vi "Set Metadata.vi"(8 "error in (no error)":errorcluster, 9 "Sphere Indicator":T5=enum."Insulated Sphere", 10 "Analyzer Choice":T3, 11 "Instrument Control \nSwitches":T4) -> (0 "error out":errorcluster, 2 "Metadata Cluster Out":T2)   [LabVIEW 2014, in "Metadata.lvlib"]
uses:
  Metadata.lvlib
  avantesSpectrometer/Acquisition/Sphere Indicator.ctl
  controls/Instrument Control Switches.ctl
  controls/Analyzer Choice.ctl
  Metadata Control.ctl
  Metadata Cluster.ctl
  avantesSpectrometer/AvaSpec.lvlib
panel:
  in  "Tab Control":enum32{"Naked Sphere", "Insulated Sphere"}(tab)
  in  "Metadata Fields Naked Sphere":T1
  in  "Metadata Fields Insualted Sphere":T1
  in  "Output Path":path
  in  "Cancel":bool
  in  "Ready?":bool
  # "Fill out the follow data fields for each test. An error will be thrown if any data fields are missing.\nNew parameters for data fields can be added by right clicking, hitting \"properties\", then \"edit items\""
  # "Off screen"
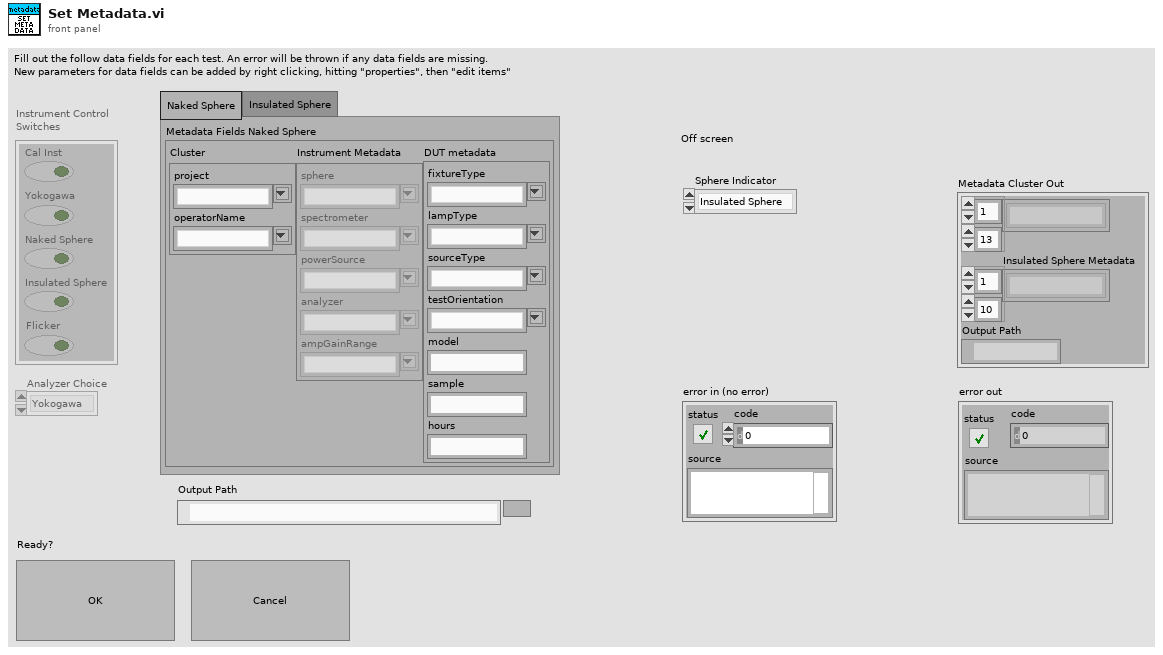
[diagram p1: front panel]
types:
  T1 = typedef "Metadata Control.ctl" = cluster{"Cluster":cluster{"project":string, "operatorName":string}, "Instrument Metadata":cluster{"sphere":string, "spectrometer":string, "powerSource":string, "analyzer":string, "ampGainRange":string}, "DUT metadata":cluster{"fixtureType":string, "lampType":string, "sourceType":string, "testOrientation":string, "model":string, "sample":string, "hours":string}}
  T2 = typedef "Metadata Cluster.ctl" = cluster{"Naked Sphere Metadata":string[][], "Insulated Sphere Metadata":string[][], "Output Path":path}
  T3 = typedef "Analyzer Choice.ctl" = enum16{"Yokogawa", "Cal Inst"}
  T4 = typedef "Instrument Control Switches.ctl" = cluster{"Cal Inst":bool, "Yokogawa":bool, "Naked Sphere":bool, "Insulated Sphere":bool, "Flicker":bool}
  T5 = typedef "AvaSpec.lvlib/Sphere Indicator.ctl" = enum16{"Naked Sphere", "Insulated Sphere"}
  T6 = enum8{"Enabled", "Disabled", "Disabled and Grayed Out"}
  T7 = cluster{"sphere":string, "spectrometer":string, "powerSource":string, "analyzer":string, "ampGainRange":string}
  T8 = cluster{"fixtureType":string, "lampType":string, "sourceType":string, "testOrientation":string, "model":string, "sample":string, "hours":string}
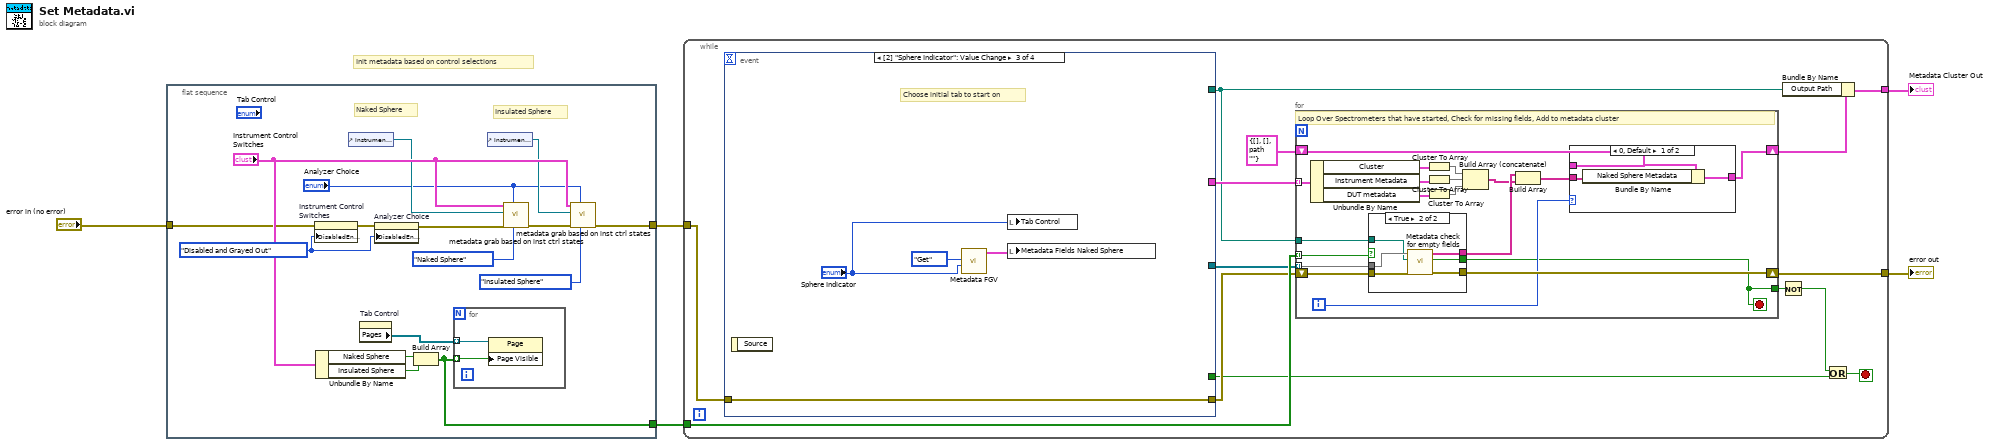
[diagram p0: block diagram]
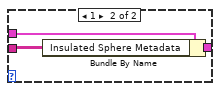
[diagram p2: hidden frame]
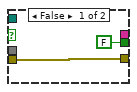
[diagram p3: hidden frame]
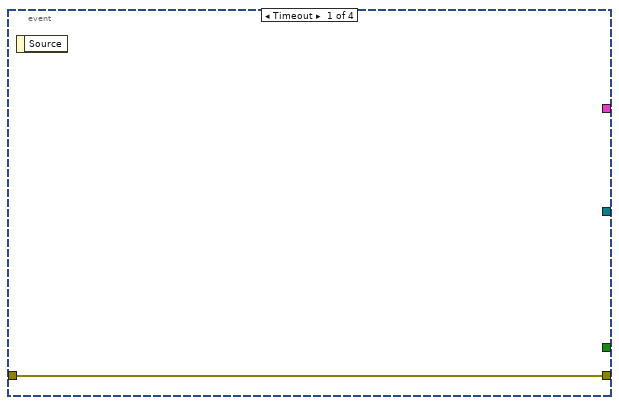
[diagram p4: hidden frame]
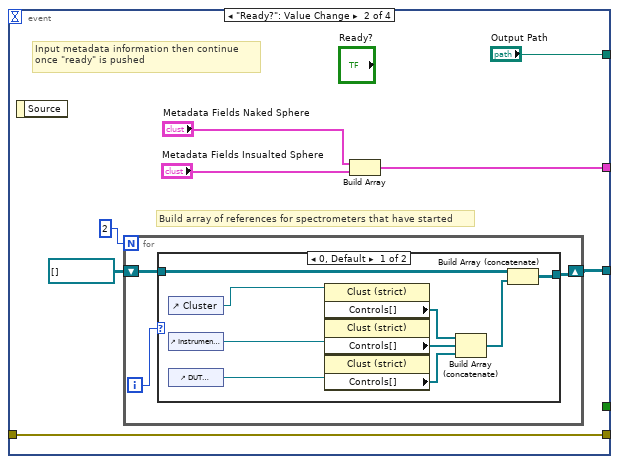
[diagram p5: hidden frame]
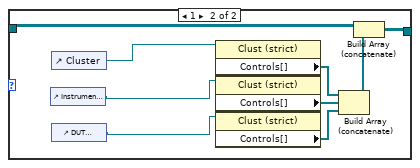
[diagram p6: hidden frame]
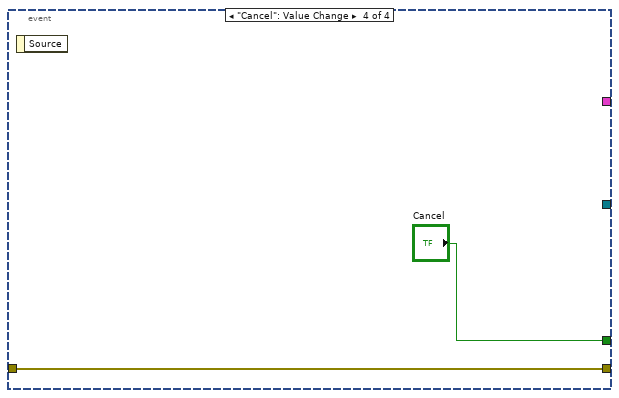
[diagram p7: hidden frame]
diagram:
  # "Init metadata based on control selections"
  n1 = flat-sequence {
    tunnel: [w20] -> w4
    tunnel: [w13] -> w3
    tunnel: "error in (no error)" -> [w9]
    frame #0 {
      w6 = T6."Disabled and Grayed Out" ("Disabled")
      # "Insulated Sphere"
      # "Naked Sphere"
      n2 = property on="Instrument Control \nSwitches" class="Clust (strict)"(error in=w9, "DisabledEnum"=w6) -> (error out=w8:errorcluster)  [unwired: 1 in, 1 out]
      n3 = Unbundle By Name("Instrument Control \nSwitches") -> ("Naked Sphere"=w16:bool, "Insulated Sphere"=w15:bool)
      n4 = control-ref of="Instrument Metadata"() -> (w12:refnum<vi>)
      n5 = property on="Tab Control" class="TabCtl (strict)"() -> ("Pages"=w14:refnum<vi>[])  [unwired: 2 in, 2 out]
      n6 = property on="Analyzer Choice" class="Enum (strict)"(error in=w8, "DisabledEnum"=w6) -> (error out=w7:errorcluster)  [unwired: 1 in, 1 out]
      n7 = Build Array(w16, w15) -> (w13:bool[])
      n8 = for {
        tunnel: w13 -> [w22] mode=indexing
        tunnel: w14 -> [w23] mode=indexing
        n9 = property class="Page"(reference=w23, "Page Visible"=w22) -> ()  [unwired: 1 in, 2 out]
      }
      n10 = control-ref of="Instrument Metadata"() -> (w11:refnum<vi>)
      n11 = call "metadata grab based on inst ctrl states.vi"("Sphere Indicator"=Sphere_Indicator."Naked Sphere" ("Sphere Indicator 2"), "Analyzer Choice"="Analyzer Choice", "error in (no error)"=w7, "Instrument Metadata"=w12, "Instrument Control \nSwitches"="Instrument Control \nSwitches") -> ("error out"=w21:errorcluster)  [unwired: 6 in]
      n12 = call "metadata grab based on inst ctrl states.vi"("Sphere Indicator"=Sphere_Indicator."Insulated Sphere" ("Sphere Indicator 2"), "Analyzer Choice"="Analyzer Choice", "error in (no error)"=w21, "Instrument Metadata"=w11, "Instrument Control \nSwitches"="Instrument Control \nSwitches") -> ("error out"=w20:errorcluster)  [unwired: 6 in]
    }
  }
  n13 = while {
    tunnel: w4 -> [w37]
    tunnel: [w36] -> w1
    tunnel: w3 -> [w34]
    tunnel: [w29] -> w2
    stop <- w35 stop-if-true
    n14 = event shown="[2] \"Sphere Indicator\": Value Change" {
      selector: _ -> [_ _ _ _]
      dyn-events: _ -> [_ _ _ _]
      timeout: _ -> [_ _ _ _]
      tunnel: w37 -> [w71 w72 w102 w106]
      tunnel: [w71 w72 w102 w106] -> w31
      tunnel: [_ _ _ "Cancel"] -> w28
      tunnel: [_ "Output Path" _ _] -> w25
      tunnel: [_ w78 _ _] -> w32
      tunnel: [_ w74 _ _] -> w33
      event Timeout {
        n15 = event-data() -> ()  [unwired: 1 in, 1 out]
      }
      event "Ready?": Value Change {
        # "Build array of references for spectrometers that have started"
        # "Input metadata information then continue\nonce \"ready\" is pushed"
        n16 = event-data() -> ()  [unwired: 1 in, 1 out]
        n17 = for {
          N: 2 -> [_]
          shift-right: [w80] -> w78
          shift-left: refnum<vi>[][] [] -> [w81]
          i -> [w82]
          n18 = case shown="0, Default" w82 {
            tunnel: [w84 w93] -> w80
            tunnel: w81 -> [w83 w92]
            frame 0, Default {
              n19 = control-ref of="Cluster"() -> (w88:refnum<vi>)
              n20 = control-ref of="Instrument Metadata"() -> (w87:refnum<vi>)
              n21 = control-ref of="DUT metadata"() -> (w86:refnum<vi>)
              n22 = property class="Clust (strict)"(reference=w88) -> ("Controls[]"=w91:refnum<vi>[])  [unwired: 1 in, 2 out]
              n23 = property class="Clust (strict)"(reference=w87) -> ("Controls[]"=w90:refnum<vi>[])  [unwired: 1 in, 2 out]
              n24 = property class="Clust (strict)"(reference=w86) -> ("Controls[]"=w89:refnum<vi>[])  [unwired: 1 in, 2 out]
              n25 = Build Array (concatenate)(w91, w90, w89) -> (w85:refnum<vi>[])
              n26 = Build Array (concatenate)(w83, w85) -> (w84:refnum<vi>[][])
            }
            frame 1 {
              n27 = control-ref of="Instrument Metadata"() -> (w95:refnum<vi>)
              n28 = control-ref of="Cluster"() -> (w96:refnum<vi>)
              n29 = control-ref of="DUT metadata"() -> (w94:refnum<vi>)
              n30 = property class="Clust (strict)"(reference=w96) -> ("Controls[]"=w100:refnum<vi>[])  [unwired: 1 in, 2 out]
              n31 = property class="Clust (strict)"(reference=w95) -> ("Controls[]"=w99:refnum<vi>[])  [unwired: 1 in, 2 out]
              n32 = property class="Clust (strict)"(reference=w94) -> ("Controls[]"=w98:refnum<vi>[])  [unwired: 1 in, 2 out]
              n33 = Build Array (concatenate)(w100, w99, w98) -> (w97:refnum<vi>[])
              n34 = Build Array (concatenate)(w92, w97) -> (w93:refnum<vi>[][])
            }
          }
        }
        n35 = Build Array("Metadata Fields Naked Sphere", "Metadata Fields Insualted Sphere") -> (w74:T1[])
      }
      event Value Change {
        # "Choose initial tab to start on"
        n36 = event-data() -> ()  [unwired: 1 in, 1 out]
        n37 = call "Metadata FGV.vi"("Sphere Indicator"="Sphere Indicator", "Control"=enum16{"Get", "Set"}."Get") -> ("Metadata Fields Out"=w103:T1)  [unwired: 9 in]
        n38 = local write "Tab Control"("Sphere Indicator") -> ()
        n39 = local write "Metadata Fields Naked Sphere"(w103) -> ()
      }
      event "Cancel": Value Change {
        n40 = event-data() -> ()  [unwired: 1 in, 1 out]
      }
    }
    n41 = for {
      tunnel: w34 -> [w55] mode=indexing
      tunnel: w33 -> [w47] mode=indexing
      tunnel: w32 -> [w54] mode=indexing
      shift-right: [w42] -> w30
      shift-left: T2 {"Naked Sphere Metadata"=[], "Insulated Sphere Metadata"=[], "Output Path"=path ""} ("Metadata Cluster Out 2") -> [w39]
      shift-right: [w56] -> w36
      shift-left: w31 -> [w41]
      tunnel: [w40] -> w27
      tunnel: w25 -> [w38]
      i -> [w46]
      stop <- w40 stop-if-true
      # "Loop Over Spectrometers that have started, Check for missing fields, Add to metadata cluster"
      n42 = Unbundle By Name(w47) -> ("Cluster"=w53:cluster{"project":string, "operatorName":string}, "Instrument Metadata"=w51:T7, "DUT metadata"=w50:T8)
      n43 = case shown="True" w55 {
        tunnel: [_ w70] -> w44
        tunnel: w41 -> [w63 w69]
        tunnel: [w63 w68] -> w56
        tunnel: [FALSE ("Missing Field") w67] -> w40
        tunnel: w54 -> [_ w66]
        tunnel: w38 -> [_ w65]
        frame False {
        }
        frame True {
          n44 = call "Metadata check for empty fields.vi"("error in (no error)"=w69, "Output Path"=w65, "Control references"=w66) -> ("error out"=w68:errorcluster, "Missing Field"=w67:bool, "Field Names"=w70:string[])  [unwired: 6 in]
        }
      }
      n45 = Cluster To Array(cluster=w53) -> (array=w52:string[])
      n46 = Cluster To Array(cluster=w51) -> (array=w49:string[])
      n47 = Cluster To Array(cluster=w50) -> (array=w48:string[])
      n48 = Build Array (concatenate)(w52, w49, w48) -> (w43:string[])
      n49 = Build Array(w44, w43) -> (w45:string[][])
      n50 = case shown="0, Default" w46 {
        tunnel: w39 -> [w59 w62]
        tunnel: w45 -> [w57 w60]
        tunnel: [w58 w61] -> w42
        frame 0, Default {
          n51 = Bundle By Name(cluster=w59, "Naked Sphere Metadata"=w57) -> (w58:T2)
        }
        frame 1 {
          n52 = Bundle By Name(cluster=w62, "Insulated Sphere Metadata"=w60) -> (w61:T2)
        }
      }
    }
    n53 = Not(x=w27) -> (.not. x?=w26:bool)
    n54 = Bundle By Name(cluster=w30, "Output Path"=w25) -> (w29:T2)
    n55 = Or(x=w26, y=w28) -> (x .or. y?=w35:bool)
  }
  "error out" <- w1
  "Metadata Cluster Out" <- w2
